vi "toggleSwitch.vi"(11 "Button":bool) -> (3 "State":bool)   [LabVIEW 2016]
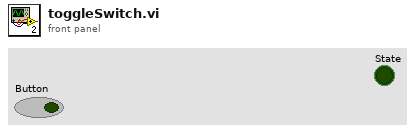
[diagram p1: front panel]
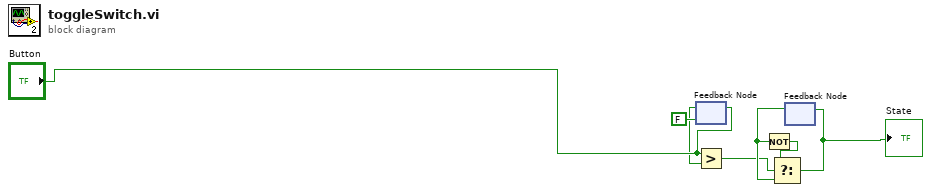
[diagram p0: block diagram]
diagram:
  n1 = feedback #1(FALSE) -> (w2:bool)
  n2 = feedback-in #1("Button") -> ()
  n3 = Greater?(x="Button", y=w2) -> (0:w5:bool)
  n4 = feedback #2() -> (w7:bool)  [unwired: 1 in]
  n5 = Not(x=w7) -> (.not. x?=w6:bool)
  n6 = Select(t=w6, s=w5, f=w7) -> (s? t:f=w1:bool)
  "State" <- w1
  n7 = feedback-in #2(w1) -> ()
